vi "Get Picture.vi"(8 "error in (no error)":errorcluster, 11 "Plastic in":refnum<class "Plastic.lvclass">) -> (0 "error out":errorcluster, 2 "Picture":picture, 3 "Plastic out":refnum<class "Plastic.lvclass">)   [LabVIEW 2020, in "Plastic.lvclass"]
uses:
  Plastic.lvclass
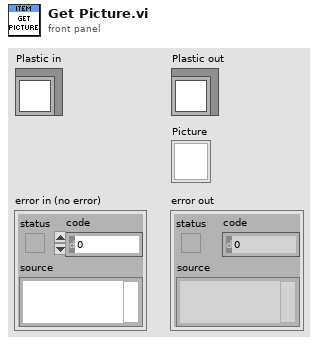
[diagram p1: front panel]
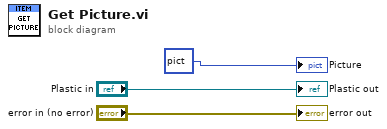
[diagram p0: block diagram]
diagram:
  "error out" <- "error in (no error)"
  "Plastic out" <- "Plastic in"
  "Picture" <- picture bytes[3230] ("new picture")
